vi "testCam.vi"() -> ()   [LabVIEW 2011]
uses:
  shared/OnOffTypeDef.ctl
  <vilib>/userdefined/High Color/IMAQdx.ctl
  <vilib>/vision/driver/NI_Vision_Acquisition_Software.lvlib
  Program Files/National Instruments/LabVIEW 2011/resource/objmgr/imaqdx.rc
  <vilib>/vision/NI_Vision_Development_Module.lvlib
panel:
  out "code":i32
  in  "Wait for trigger":bool=TRUE
  in  "stop":bool
  out "Image Dst Out":T1(plugin-control)
  out "Acquisition OK?":bool
  in  "error in":errorcluster
  in  "x":T2
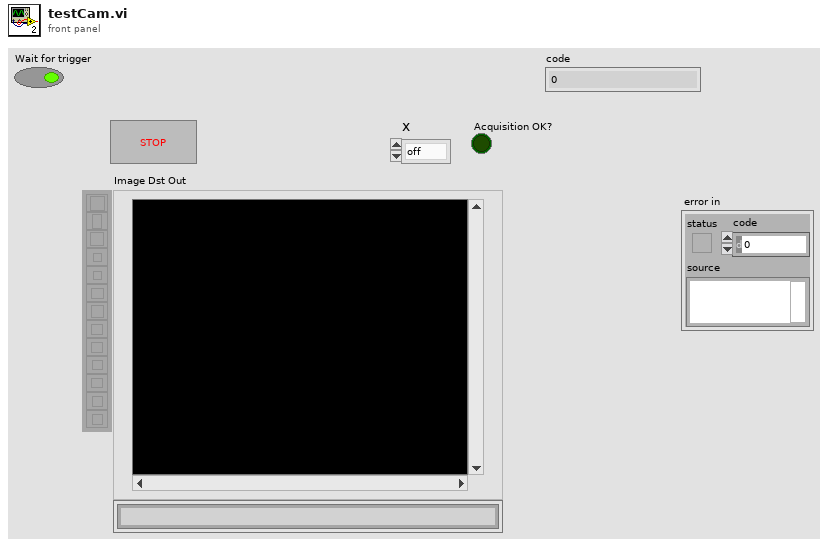
[diagram p1: front panel]
types:
  T1 = typedef "IMAQ Image.ctl" = refnum<image>
  T2 = typedef "OnOffTypeDef.ctl" = enum16{"off", "on"}
  T3 = typedef "Image Type" = u32
  T4 = typedef "IMAQdx.ctl" = refnum<k21>
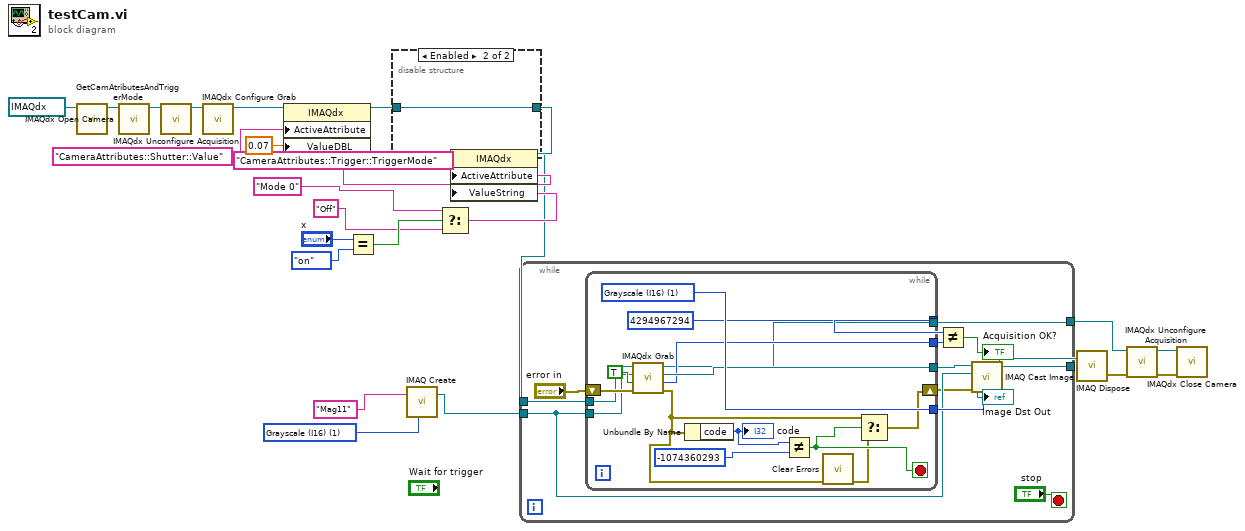
[diagram p0: block diagram]
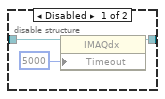
[diagram p2: hidden frame]
diagram:
  w18 = T3 1 items=["Grayscale (U8)", "Grayscale (I16)", "Grayscale (SGL)", "Complex (CSG)", "RGB (U32)", "HSL (U32)", "RGB (U64)", "Grayscale (U16)"] ("Image Type")
  n1 = call "GetCamAtributesAndTriggerMode.vi"("IMAQdx Session"=T4 "cam1") -> ("IMAQdx Session 2"=w21:T4)  [unwired: 7 in, 3 out]
  n2 = call <vilib>:"IMAQdx Open Camera.vi"("Session In"=w21) -> ("Session Out"=w22:T4)  [unwired: 2 in, 8 out]
  n3 = call <vilib>:"IMAQdx Unconfigure Acquisition.vi"("Session In"=w22) -> ("Session Out"=w23:T4)  [unwired: 1 in, 9 out]
  n4 = call <vilib>:"IMAQdx Configure Grab.vi"("Session In"=w23) -> ("Session Out"=w24:T4)  [unwired: 1 in, 9 out]
  n5 = property class="IMAQdx"(reference=w24, "ActiveAttribute"="CameraAttributes::Shutter::Value", "ValueDBL"=0.07) -> (reference out=w12:T4)  [unwired: 1 in, 1 out]
  n6 = Equal?(x="x", y=OnOffTypeDef."on" ("Save")) -> (x = y?=w15:bool)
  n7 = disable-structure shown="Enabled" {
    disable-tunnel: w12 -> [w27 w29]
    disable-tunnel: [w26 w29] -> w11
    frame Disabled {
      n8 = property class="IMAQdx"(reference=w27, "Timeout"=u32 5000) -> (reference out=w26:T4)  [unwired: 1 in, 1 out]
    }
    frame Enabled {
    }
  }
  n9 = call "IMAQ Create"("Image Name"="Mag11", "Image Type"=w18) -> ("New Image"=w7:T1)  [unwired: 3 in, 1 out]
  n10 = Select(t="Mode 0", s=w15, f="Off") -> (s? t:f=w9:string)
  n11 = property class="IMAQdx"(reference=w11, "ActiveAttribute"="CameraAttributes::Trigger::TriggerMode", "ValueString"=w9) -> (reference out=w6:T4)  [unwired: 1 in, 1 out]
  n12 = while {
    tunnel: w7 -> [w38]
    tunnel: w6 -> [w37]
    tunnel: [w33] -> w2
    tunnel: [w32] -> w1
    stop <- "stop" stop-if-true
    n13 = while {
      tunnel: [w55] -> w41
      tunnel: [w54] -> w40
      tunnel: w38 -> [w52]
      tunnel: w37 -> [w51]
      tunnel: [u32 4294967294 ("Buffer Number Out")] -> w36
      tunnel: [w49] -> w34
      tunnel: [w48] -> w32
      shift-right: [w42] -> w30
      shift-left: "error in" -> [w53]
      stop <- w45 stop-if-true
      w55 = T3 1 items=["Grayscale (U8)", "Grayscale (I16)", "Grayscale (SGL)", "Complex (CSG)", "RGB (U32)", "HSL (U32)", "RGB (U64)", "Grayscale (U16)"] ("Image Type")
      n14 = call <vilib>:"IMAQdx Grab.vi"("error in"=w53, "Wait for Next Buffer? (Yes)"=TRUE, "Image In"=w52, "Session In"=w51) -> ("error out"=w44:errorcluster, "Buffer Number Out"=w49:u32, "Image Out"=w54:T1, "Session Out"=w48:T4)  [unwired: 4 out]
      n15 = Unbundle By Name(w44) -> ("code"=w47:i32)
      "code" <- w47
      n16 = Not Equal?(x=w47, y=-1074360293 ("code 2")) -> (x != y?=w45:bool)
      n17 = call <vilib>:"Clear Errors.vi"("error in (no error)"=w44) -> ("error out"=w43:errorcluster)  [unwired: 6 in]
      n18 = Select(t=w44, s=w45, f=w43) -> (s? t:f=w42:errorcluster)
    }
    n19 = Not Equal?(x=w36, y=w34) -> (x != y?=→"Acquisition OK?":bool)
    n20 = call "IMAQ Cast Image"("Image Type"=w41, "error in (no error)"=w30, "Image Dst"=w38, "Image Src"=w40) -> ("Image Dst Out"=w33:T1)  [unwired: 6 in, 1 out]
    "Image Dst Out" <- w33
  }
  n21 = call "IMAQ Dispose"("Image"=w2) -> ("error out"=w5:errorcluster)  [unwired: 5 in]
  n22 = call <vilib>:"IMAQdx Unconfigure Acquisition.vi"("error in"=w5, "Session In"=w1) -> ("error out"=w3:errorcluster, "Session Out"=w4:T4)  [unwired: 8 in]
  n23 = call <vilib>:"IMAQdx Close Camera.vi"("error in"=w3, "Session In"=w4) -> ()  [unwired: 9 in, 1 out]
